vi "Create User UI.vi"() -> ()   [LabVIEW 2016, in "LV-Data.PGSQL.lvclass"]
uses:
  LV-Data.PGSQL.lvclass
  LV-Data/Typedefs/Operation--enum.ctl
  <userlib>/_OpenG.lib/numeric/numeric.llb/Random Number Within Range - DBL__ogtk.vi
  <vilib>/ErrorRing/Error Ring.xnode
  LV-Data/LV-Data.lvclass
panel:
  in  "Delete Permission":bool
  out "Selected User (inst)":string
  in  "Permissions":i32(listbox)
  in  "Give data write permission":bool
  in  "Delete user (inst)":bool
  in  "Users":i32(listbox)
  out "new password":string
  out "new user (inst) name":string
  in  "path to object in table":string
  in  "new password":string
  in  "Create user (inst)":bool
  in  "generate random password?":bool
  in  "new user (inst) name":string
  in  "STOP":bool
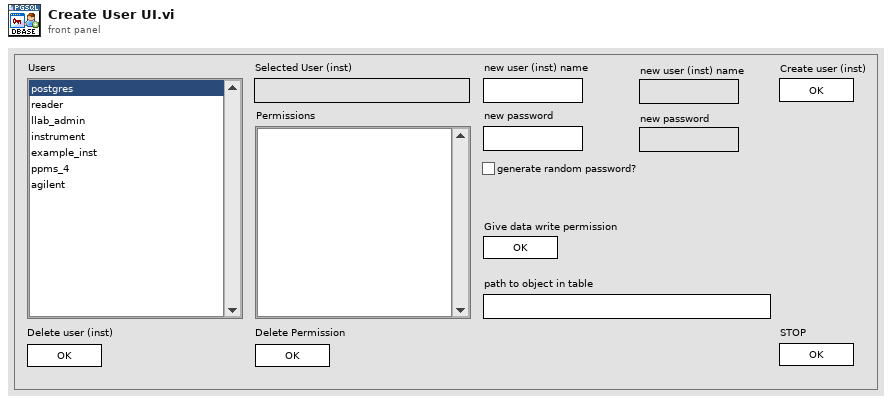
[diagram p1: front panel]
types:
  T1 = enum32{"Invalid", "Standard", "Closed", "Hidden", "Minimized", "Maximized"}
  T2 = enum32{"invalid app kind", "Development System", "Run Time System", "Student Edition", "Embedded LabVIEW", "Evaluation", "Custom"}
  T3 = typedef "LV-Data.lvclass/Operation--enum.ctl" = enum16{"Read", "Write", "Write + Append"}
  T4 = cluster{"Core":cluster{"Current VI Reference":refnum<vi>, "Close Panel on Exit?":bool}, "user":string, "password":string, "path to something in table":string, "new instrument name":string, "names already taken":string[], "Data.PG":refnum<class "LV-Data.PGSQL.lvclass">, "Selected instrument":string, "Selected inst privileges":string[], "Selected inst privileges names":string[], "Selected privilege":string}
  T5 = cluster{"Current VI Reference":refnum<vi>, "Close Panel on Exit?":bool}
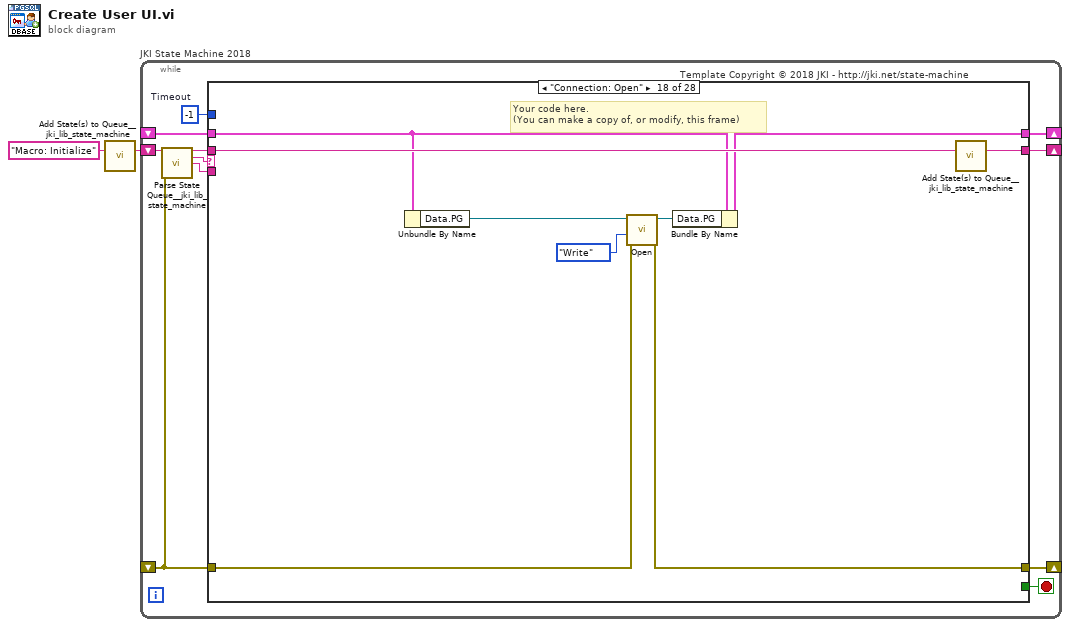
[diagram p0: block diagram]
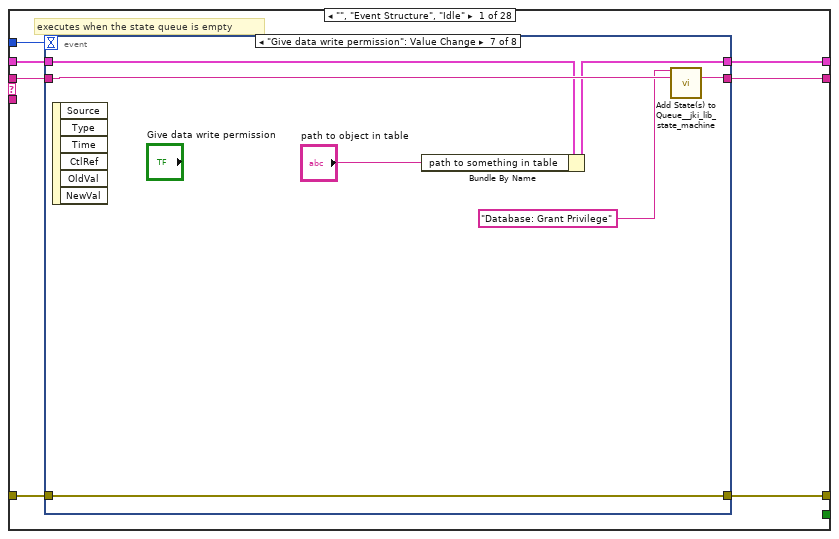
[diagram p2: hidden frame]
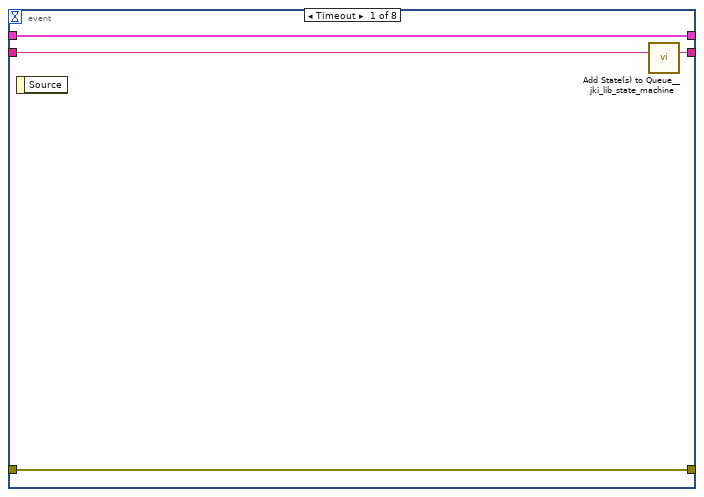
[diagram p3: hidden frame]
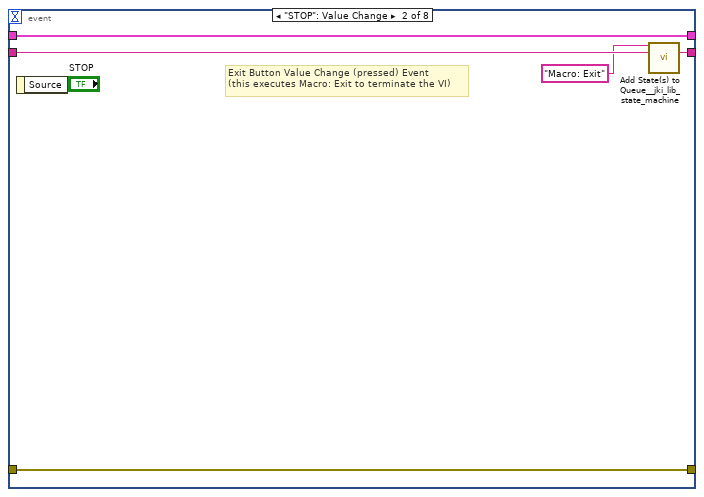
[diagram p4: hidden frame]
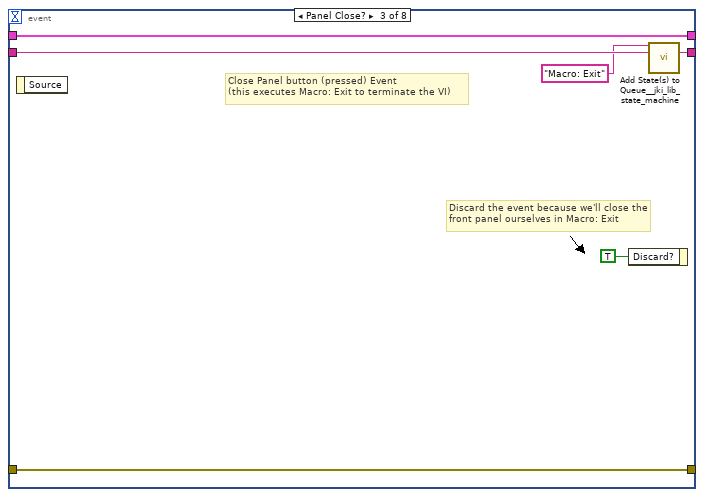
[diagram p5: hidden frame]
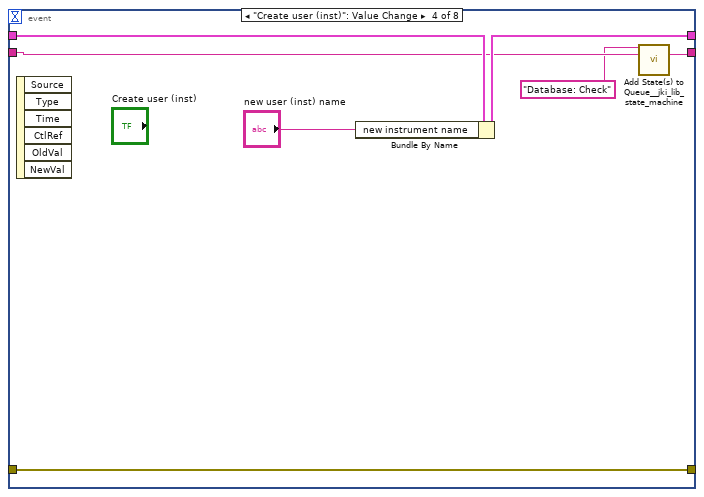
[diagram p6: hidden frame]
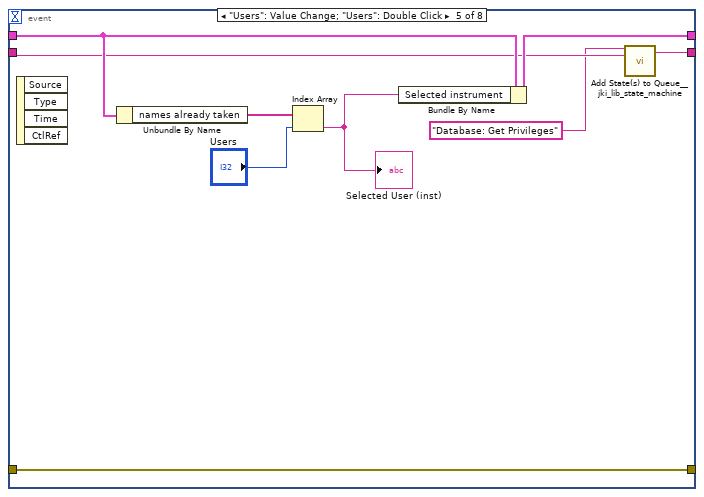
[diagram p7: hidden frame]
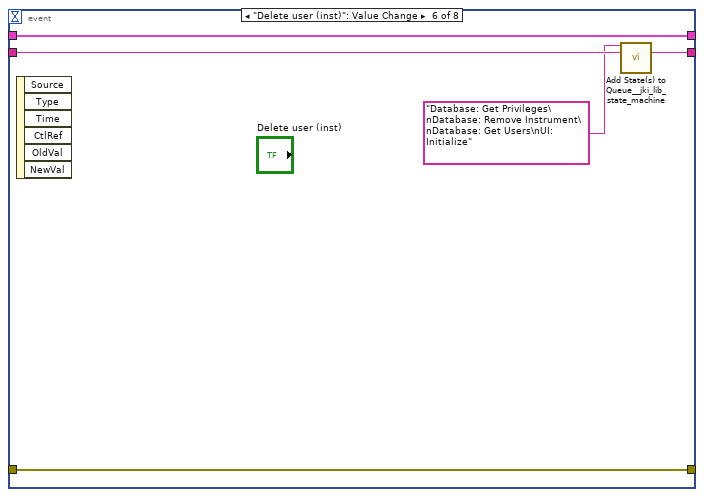
[diagram p8: hidden frame]
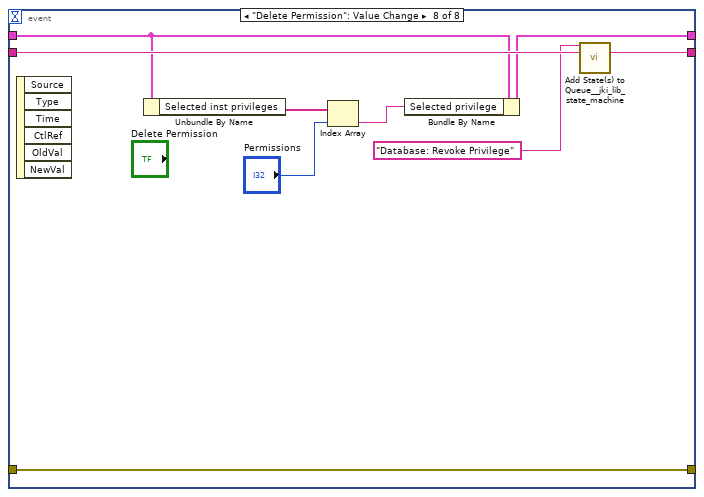
[diagram p9: hidden frame]
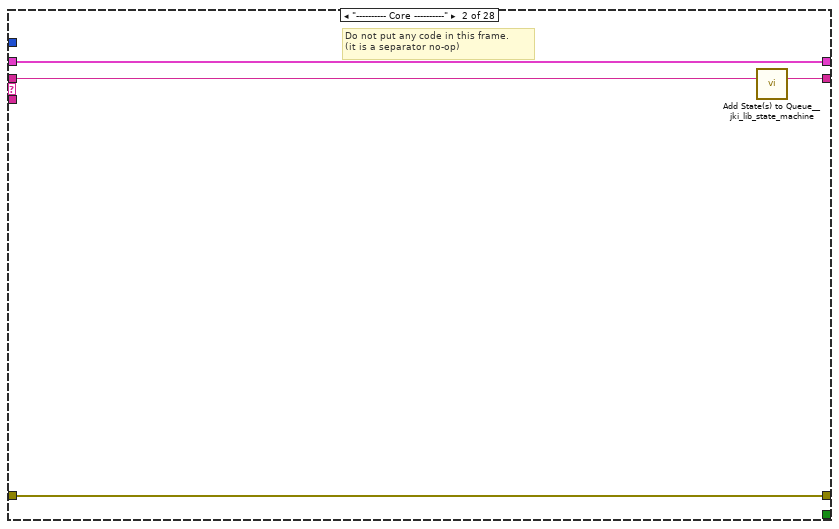
[diagram p10: hidden frame]
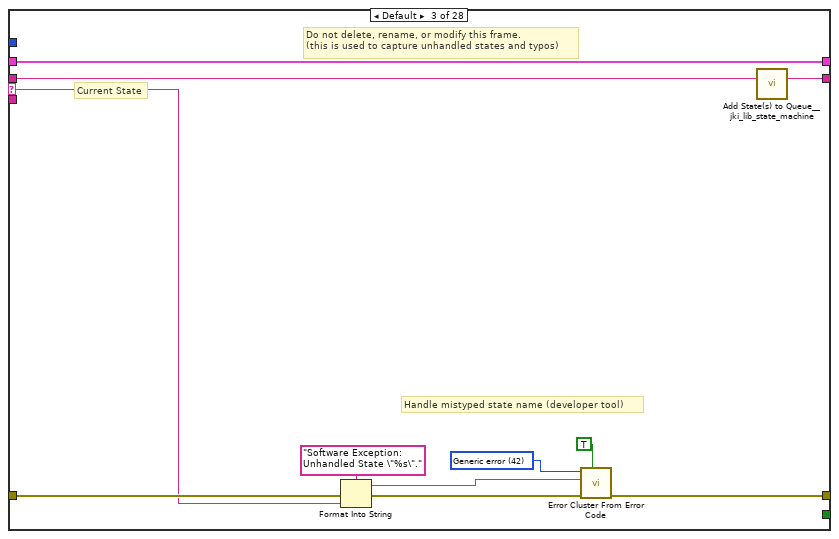
[diagram p11: hidden frame]
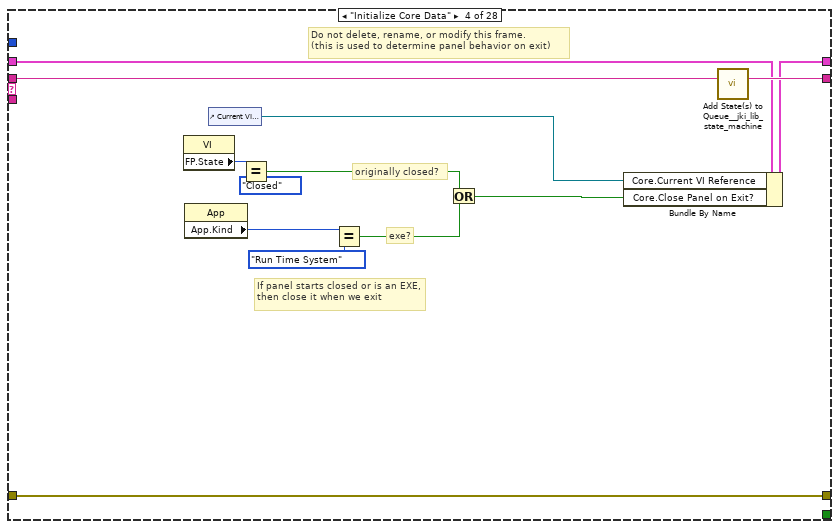
[diagram p12: hidden frame]
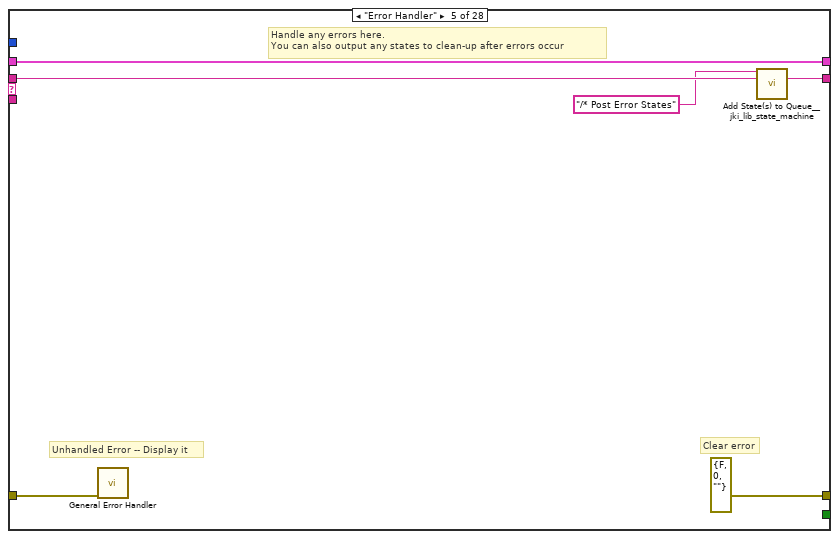
[diagram p13: hidden frame]
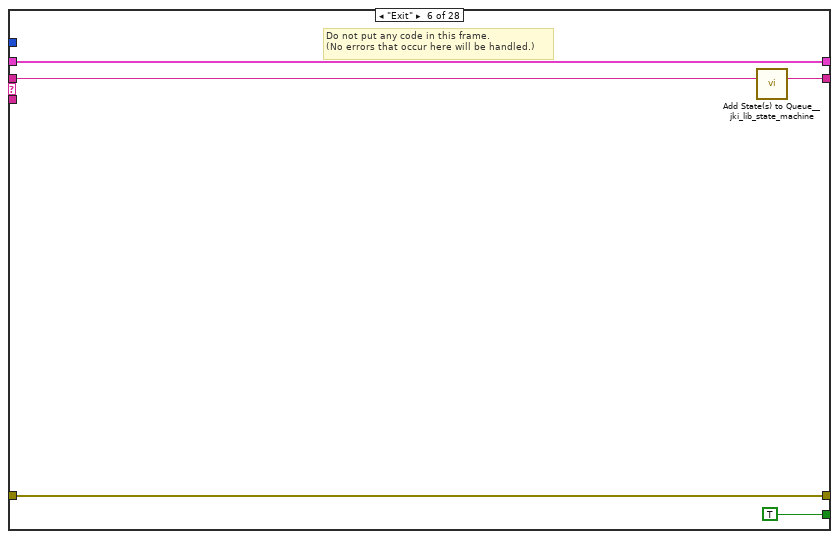
[diagram p14: hidden frame]
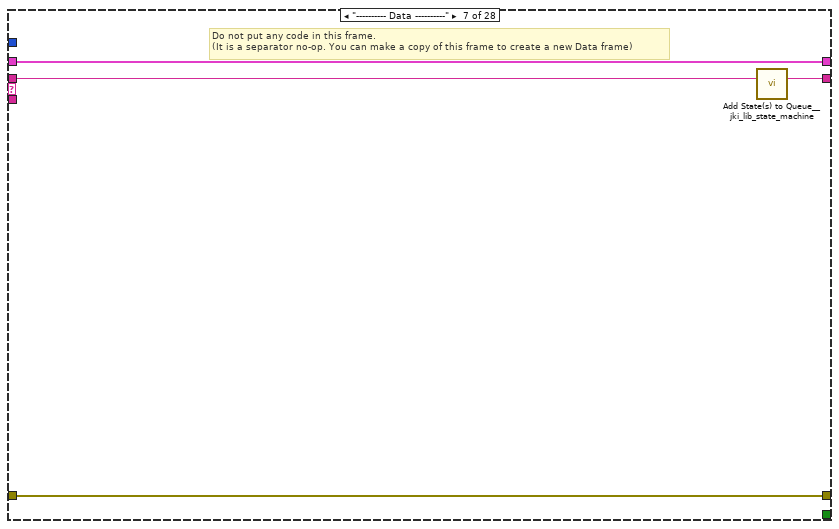
[diagram p15: hidden frame]
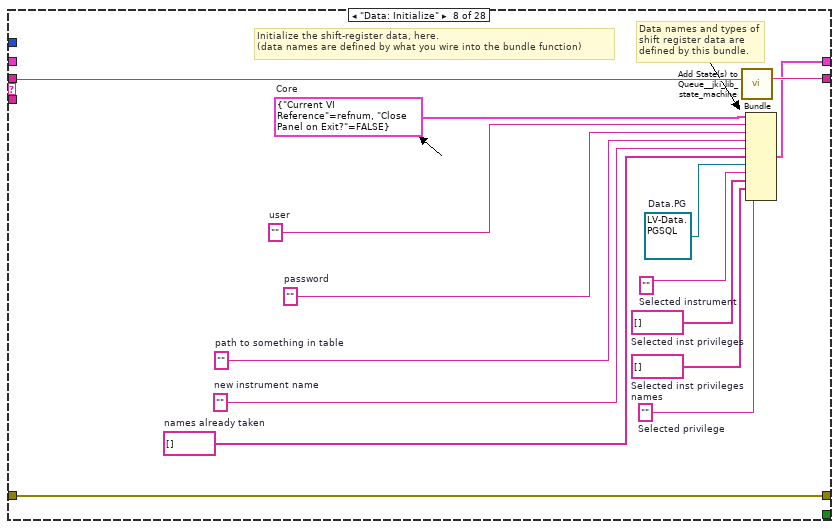
[diagram p16: hidden frame]
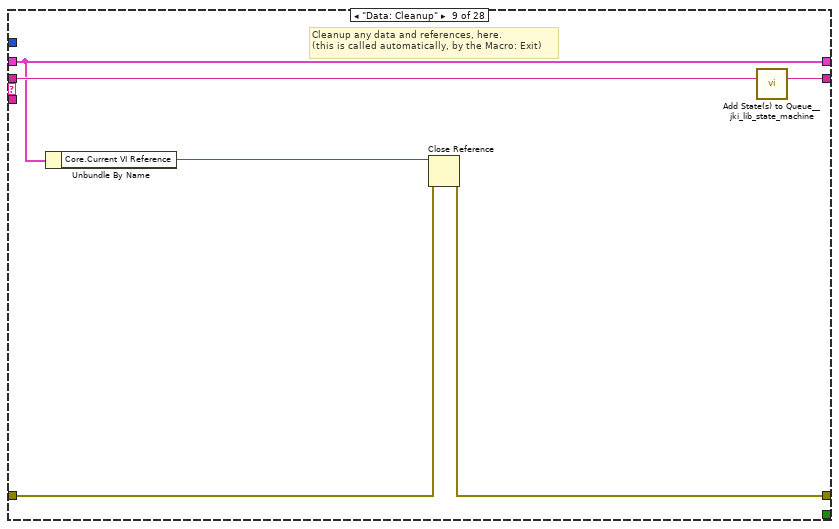
[diagram p17: hidden frame]
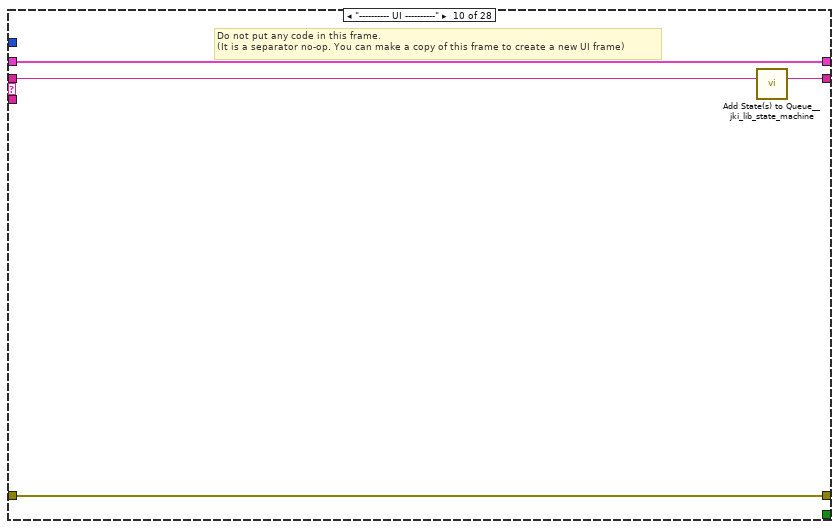
[diagram p18: hidden frame]
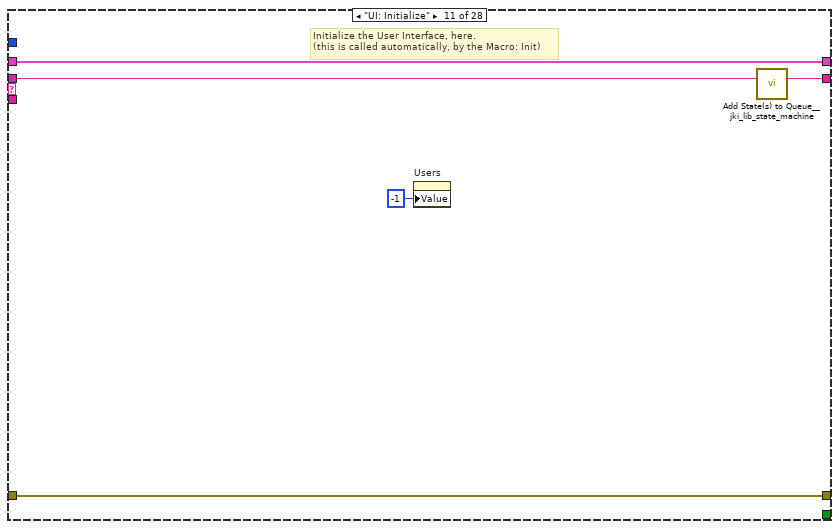
[diagram p19: hidden frame]
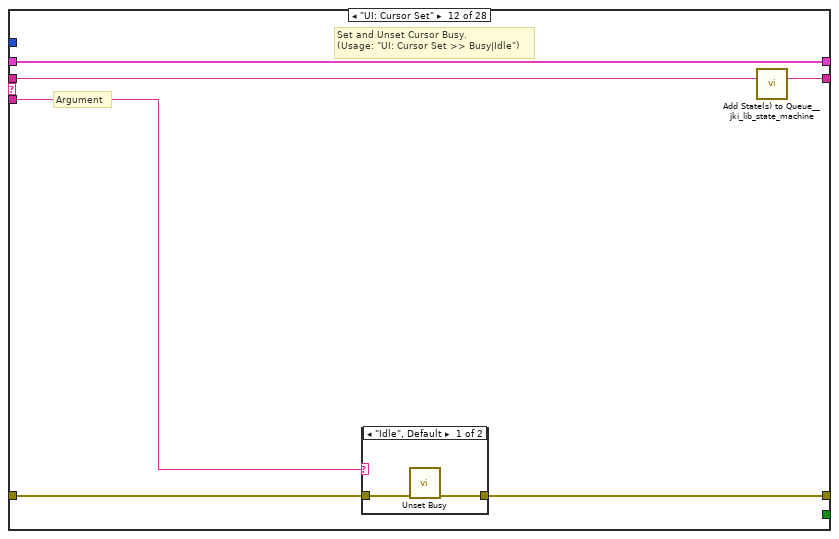
[diagram p20: hidden frame]
diagram:
  n1 = call <vilib>:"Add State(s) to Queue__jki_lib_state_machine.vi"("State(s) in (\"\")"="Macro: Initialize") -> ("States Out"=w2:string)  [unwired: 14 in]
  n2 = while "JKI State Machine 2018" {
    shift-right: [w6] -> _
    shift-left: _ -> [w5]
    shift-right: [w9] -> _
    shift-left: _ -> [w3]
    shift-right: [w8] -> _
    shift-left: w2 -> [w10]
    stop <- w7 stop-if-true
    w4 = -1  # Timeout
    # "Template Copyright © 2018 JKI - http://jki.net/state-machine"
    n3 = call <vilib>:"Parse State Queue__jki_lib_state_machine.vi"("State Queue"=w10, "Error In (no error)"=w3) -> ("Remaining States"=w12:string, "Current State"=w13:string, "Arguments"=w11:string)  [unwired: 11 in]
    n4 = case shown="\"Connection: Open\"" w13 {
      selector: w13 -> [_ _ w77 _ _ _ _ _ _ _ _ _ _ _ _ _ _ _ _ _ _ _ _ _ _ _ _ _]
      tunnel: w12 -> [w20 w76 w81 w100 w106 w111 w115 w130 w136 w140 w145 w151 w162 w231 w236 w247 w251 w260 w266 w270 w279 w291 w326 w340 w353 w368 w378 w408]
      tunnel: w11 -> [_ _ _ _ _ _ _ _ _ _ _ w146 w156 _ _ _ _ _ _ _ _ _ _ _ _ _ _ _]
      tunnel: w5 -> [w18 w73 w79 w93 w103 w109 w112 _ w131 w137 w143 w149 w158 w228 w233 w244 w248 w257 w264 w267 w272 w283 w314 w330 w344 w362 w370 w402]
      tunnel: [w17 w74 w83 w97 errorcluster {"status"=FALSE, "code"=0, "source"=""} ("error out") w108 w113 w128 w132 w138 w142 w147 w159 w229 w234 w245 w249 w253 w261 w268 w274 w281 w322 w337 w345 w354 w372 w399] -> w9
      tunnel: w3 -> [w16 w74 w82 w97 w102 w108 w113 w128 w133 w138 w142 w148 w160 w229 w234 w245 w249 w254 w262 w268 w275 _ w321 w338 w346 w355 w371 w403]
      tunnel: [w19 w75 w80 w99 w105 w110 w114 w129 w135 w139 w144 w150 w161 w230 w235 w246 w250 w259 w265 w269 w278 w290 w325 w339 w352 w367 w377 w407] -> w8
      tunnel: [_ _ _ _ _ TRUE _ _ _ _ _ _ _ _ _ _ _ _ _ _ _ _ _ _ _ _ _ _] -> w7
      tunnel: [w15 w73 w79 w98 w103 w109 w112 w123 w131 w137 w143 w149 w158 w228 w233 w244 w248 w258 w264 w267 w276 w283 w313 w329 w343 w361 w369 w401] -> w6
      tunnel: w4 -> [w14 _ _ _ _ _ _ _ _ _ _ _ _ _ _ _ _ _ _ _ _ _ _ _ _ _ _ _]
      frame "", "Event Structure", "Idle" {
        # "executes when the state queue is empty"
        n5 = event shown="[6] \"Give data write permission\": Value Change" {
          selector: _ -> [_ _ _ _ _ _ _ _]
          dyn-events: _ -> [_ _ _ _ _ _ _ _]
          timeout: w14 -> [_ _ _ _ _ _ _ _]
          tunnel: w20 -> [w24 w29 w35 w38 w44 w53 w62 w71]
          tunnel: [w23 w28 w34 w39 w45 w54 w63 w70] -> w19
          tunnel: w18 -> [w21 w26 w32 w42 w48 w55 w57 w65]
          tunnel: [w22 w27 w33 w37 w51 w56 w61 w72] -> w17
          tunnel: w16 -> [w22 w27 w33 w37 w51 w56 w61 w72]
          tunnel: [w21 w26 w32 w41 w47 w55 w59 w68] -> w15
          event Timeout {
            n6 = event-data() -> ()  [unwired: 1 in, 1 out]
            n7 = call <vilib>:"Add State(s) to Queue__jki_lib_state_machine.vi"("State(s) in (\"\")"=w24) -> ("States Out"=w23:string)  [unwired: 14 in]
          }
          event "STOP": Value Change {
            # "Exit Button Value Change (pressed) Event\n(this executes Macro: Exit to terminate the VI)"
            n8 = event-data() -> ()  [unwired: 1 in, 1 out]
            n9 = call <vilib>:"Add State(s) to Queue__jki_lib_state_machine.vi"("State(s) in Front (\"\")"="Macro: Exit", "State(s) in (\"\")"=w29) -> ("States Out"=w28:string)  [unwired: 13 in]
          }
          event Panel Close? {
            # "Discard the event because we'll close the front panel ourselves in Macro: Exit"
            # "Close Panel button (pressed) Event\n(this executes Macro: Exit to terminate the VI)"
            n10 = event-data() -> ()  [unwired: 1 in, 1 out]
            n11 = event-data("Discard?"=TRUE) -> ()  [unwired: 1 in, 1 out]
            n12 = call <vilib>:"Add State(s) to Queue__jki_lib_state_machine.vi"("State(s) in Front (\"\")"="Macro: Exit", "State(s) in (\"\")"=w35) -> ("States Out"=w34:string)  [unwired: 13 in]
          }
          event "Create user (inst)": Value Change {
            n13 = event-data() -> ()  [unwired: 1 in, 6 out]
            n14 = Bundle By Name(cluster=w42, "new instrument name"="new user (inst) name") -> (w41:T4)
            n15 = call <vilib>:"Add State(s) to Queue__jki_lib_state_machine.vi"("State(s) in Front (\"\")"="Database: Check" ("State(s) in Front (\"\")"), "State(s) in (\"\")"=w38) -> ("States Out"=w39:string)  [unwired: 13 in]
          }
          event "Users": Value Change; "Users": Double Click {
            n16 = event-data() -> ()  [unwired: 1 in, 4 out]
            n17 = Unbundle By Name(w48) -> ("names already taken"=w50:string[])
            n18 = Index Array(array=w50, index="Users") -> (element=w46:string)
            "Selected User (inst)" <- w46
            n19 = Bundle By Name(cluster=w48, "Selected instrument"=w46) -> (w47:T4)
            n20 = call <vilib>:"Add State(s) to Queue__jki_lib_state_machine.vi"("State(s) in Front (\"\")"="Database: Get Privileges" ("State(s) in Front (\"\")"), "State(s) in (\"\")"=w44) -> ("States Out"=w45:string)  [unwired: 13 in]
          }
          event "Delete user (inst)": Value Change {
            n21 = event-data() -> ()  [unwired: 1 in, 6 out]
            n22 = call <vilib>:"Add State(s) to Queue__jki_lib_state_machine.vi"("State(s) in Front (\"\")"="Database: Get Privileges\nDatabase: Remove Instrument\nDatabase: Get Users\nUI: Initialize" ("State(s) in Front (\"\")"), "State(s) in (\"\")"=w53) -> ("States Out"=w54:string)  [unwired: 13 in]
          }
          event "Give data write permission": Value Change {
            n23 = event-data() -> ()  [unwired: 1 in, 6 out]
            n24 = Bundle By Name(cluster=w57, "path to something in table"="path to object in table") -> (w59:T4)
            n25 = call <vilib>:"Add State(s) to Queue__jki_lib_state_machine.vi"("State(s) in Front (\"\")"="Database: Grant Privilege" ("State(s) in Front (\"\")"), "State(s) in (\"\")"=w62) -> ("States Out"=w63:string)  [unwired: 13 in]
          }
          event "Delete Permission": Value Change {
            n26 = event-data() -> ()  [unwired: 1 in, 6 out]
            n27 = Unbundle By Name(w65) -> ("Selected inst privileges"=w64:string[])
            n28 = Index Array(array=w64, index="Permissions") -> (element=w67:string)
            n29 = Bundle By Name(cluster=w65, "Selected privilege"=w67) -> (w68:T4)
            n30 = call <vilib>:"Add State(s) to Queue__jki_lib_state_machine.vi"("State(s) in Front (\"\")"="Database: Revoke Privilege" ("State(s) in Front (\"\")"), "State(s) in (\"\")"=w71) -> ("States Out"=w70:string)  [unwired: 13 in]
          }
        }
      }
      frame "---------- Core ----------" {
        # "Do not put any code in this frame.\n(it is a separator no-op)"
        n31 = call <vilib>:"Add State(s) to Queue__jki_lib_state_machine.vi"("State(s) in (\"\")"=w76) -> ("States Out"=w75:string)  [unwired: 14 in]
      }
      frame Default {
        w86 = 42 items=["No error", "Argument error", "Memory is full", "Out of zone", "End of file", "File already open", "Generic file I/O error", "File not found", "File permission error", "Disk is full", "Duplicate path", "Too many files open", "System feature not enabled", "Resource file not found", "Cannot add resource", "Resource not found", "Image not found", "Image memory error", "Pen does not exist", "Config type invalid", "Config token not found", "Config parse error", "Config memory error", "Bad external code format", "Bad external code offset", "External code not present", "Null window", "Destroy window error", "Null menu", "Print aborted", "Bad print record", "Print driver error", "Windows error during printing", "Memory error during printing", "Print dialog error", "Generic print error", "Invalid device refnum", "Device not found", "Device parameter error", "Device unit error", "Cannot open device", "Device call aborted", "Generic error", "Cancelled by user", "Object ID too low", "Object ID too high", "Object not in heap", "Unknown heap", "Unknown object (invalid DefProc)", "Unknown object (DefProc not in table)", "Message out of range", "Invalid (null) method", "Unknown message", "Manager call not supported", "Bad address", "Network operation in progress", "Network operation timed out", "Connection is busy", "Network attribute not supported", "Network error", "Address in use", "System out of memory", "Connection aborted", "Connection refused", "Not connected", "Already connected", "Connection closed", "Initialization error (interapplication manager)", "Bad occurrence", "Wait on unbound occurrence handler", "Occurrence queue overflow", "Datalog type conflict", "Unused", "Unrecognized type (interapplication manager)", "Memory corrupt", "Failed to make temporary DLL", "Old CIN version", "Drag socket not found", "Failed to load drop-object", "Failed to register OLE object", "Failed to release OLE object", "Format specifier type mismatch", "Unknown format specifier", "Too few format specifiers", "Too many format specifiers", "Scan failed", "Newer CIN version", "Error converting to variant", "Runtime menu error", "Password tampered", "Variant attribute not found", "Incompatible variant data type", "Event data is not available", "Event Store is not present", "Occurrence is not found", "Event Queue is not created", "Event info is not available", "Refnum passed is NULL", "Error retrieving Class GUID", "Error retrieving CoClass GUID", "Error retrieving TypeLib GUID.", "Bad built application magic bytes.", "Specific driver is different from the specific driver associated with the Logical Name.", "There is no session opened to the class driver.", "Max Error", "MAX - Error with config objects", "MAX - Error loading configuration", "MAX - Group not supported"]
        # "Current State"
        # "Do not delete, rename, or modify this frame.\n(this is used to capture unhandled states and typos)"
        # "Handle mistyped state name (developer tool)"
        n32 = Format Into String(format string="Software Exception: Unhandled State \"%s\"." ("message"), error in=w82, w77) -> (resulting string=w85:string, error out=w84:errorcluster)  [unwired: 1 in]
        n33 = call <vilib>:"Error Cluster From Error Code.vi"("show call chain? (False)"=TRUE, "error in (no error)"=w84, "error message (\"\")"=w85, "error code (0)"=w86) -> ("error out"=w83:errorcluster)  [unwired: 5 in]
        n34 = call <vilib>:"Add State(s) to Queue__jki_lib_state_machine.vi"("State(s) in (\"\")"=w81) -> ("States Out"=w80:string)  [unwired: 14 in]
      }
      frame "Initialize Core Data" {
        # "Do not delete, rename, or modify this frame.\n(this is used to determine panel behavior on exit)"
        # "originally closed?"
        # "exe?"
        # "If panel starts closed or is an EXE, then close it when we exit"
        n35 = property class="VI"() -> ("FP.State"=w90:T1)  [unwired: 2 in, 2 out]
        n36 = property class="App"() -> ("App.Kind"=w96:T2)  [unwired: 2 in, 2 out]
        n37 = control-ref of="Current VI Reference"() -> (w91:refnum<vi>)
        n38 = Equal?(x=w90, y=T1."Closed" ("Front Panel Window:State")) -> (x = y?=w88:bool)
        n39 = Equal?(x=w96, y=T2."Run Time System" ("Application:Kind")) -> (x = y?=w94:bool)
        n40 = Or(x=w88, y=w94) -> (x .or. y?=w92:bool)
        n41 = Bundle By Name(cluster=w93, "Core.Current VI Reference"=w91, "Core.Close Panel on Exit?"=w92) -> (w98:T4)
        n42 = call <vilib>:"Add State(s) to Queue__jki_lib_state_machine.vi"("State(s) in (\"\")"=w100) -> ("States Out"=w99:string)  [unwired: 14 in]
      }
      frame "Error Handler" {
        # "Unhandled Error -- Display it"
        # "Handle any errors here.\nYou can also output any states to clean-up after errors occur"
        # "Clear error"
        n43 = call <vilib>:"General Error Handler.vi"("error in (no error)"=w102) -> ()  [unwired: 10 in, 5 out]
        n44 = call <vilib>:"Add State(s) to Queue__jki_lib_state_machine.vi"("State(s) in Front (\"\")"="/* Post Error States", "State(s) in (\"\")"=w106) -> ("States Out"=w105:string)  [unwired: 13 in]
      }
      frame "Exit" {
        # "Do not put any code in this frame.\n(No errors that occur here will be handled.)"
        n45 = call <vilib>:"Add State(s) to Queue__jki_lib_state_machine.vi"("State(s) in (\"\")"=w111) -> ("States Out"=w110:string)  [unwired: 14 in]
      }
      frame "---------- Data ----------" {
        # "Do not put any code in this frame.\n(It is a separator no-op. You can make a copy of this frame to create a new Data frame)"
        n46 = call <vilib>:"Add State(s) to Queue__jki_lib_state_machine.vi"("State(s) in (\"\")"=w115) -> ("States Out"=w114:string)  [unwired: 14 in]
      }
      frame "Data: Initialize" {
        w116 = ""  # password
        w117 = ""  # Selected privilege
        w118 = string[] []  # Selected inst privileges names
        w119 = ""  # user
        w120 = string[] []  # Selected inst privileges
        w121 = ""  # Selected instrument
        w122 = refnum<class "LV-Data.PGSQL.lvclass"> refnum  # Data.PG
        w125 = string[] []  # names already taken
        w126 = ""  # new instrument name
        w127 = ""  # path to something in table
        w124 = T5 {"Current VI Reference"=refnum, "Close Panel on Exit?"=FALSE}  # Core
        # "Data names and types of shift register data are defined by this bundle."
        # "Initialize the shift-register data, here.\n(data names are defined by what you wire into the bundle function)"
        n47 = call <vilib>:"Add State(s) to Queue__jki_lib_state_machine.vi"("State(s) in (\"\")"=w130) -> ("States Out"=w129:string)  [unwired: 14 in]
        n48 = Bundle("Core"=w124, "user"=w119, "password"=w116, "path to something in table"=w127, "new instrument name"=w126, "names already taken"=w125, "Data.PG"=w122, "Selected instrument"=w121, "Selected inst privileges"=w120, "Selected inst privileges names"=w118, "Selected privilege"=w117) -> (w123:T4)  [unwired: 1 in]
      }
      frame "Data: Cleanup" {
        # "Cleanup any data and references, here.\n(this is called automatically, by the Macro: Exit)"
        n49 = Unbundle By Name(w131) -> ("Core.Current VI Reference"=w134:refnum<vi>)
        n50 = Close Reference(reference=w134, error in (no error)=w133) -> (error out=w132:errorcluster)
        n51 = call <vilib>:"Add State(s) to Queue__jki_lib_state_machine.vi"("State(s) in (\"\")"=w136) -> ("States Out"=w135:string)  [unwired: 14 in]
      }
      frame "---------- UI ----------" {
        # "Do not put any code in this frame.\n(It is a separator no-op. You can make a copy of this frame to create a new UI frame)"
        n52 = call <vilib>:"Add State(s) to Queue__jki_lib_state_machine.vi"("State(s) in (\"\")"=w140) -> ("States Out"=w139:string)  [unwired: 14 in]
      }
      frame "UI: Initialize" {
        # "Initialize the User Interface, here.\n(this is called automatically, by the Macro: Init)"
        n53 = property on="Users" class="LstBox (strict)"("Value"=-1 ("Users")) -> ()  [unwired: 2 in, 2 out]
        n54 = call <vilib>:"Add State(s) to Queue__jki_lib_state_machine.vi"("State(s) in (\"\")"=w145) -> ("States Out"=w144:string)  [unwired: 14 in]
      }
      frame "UI: Cursor Set" {
        # "Argument"
        # "Set and Unset Cursor Busy.\n(Usage: \"UI: Cursor Set >> Busy|Idle\")"
        n55 = case shown="\"Idle\", Default" w146 {
          tunnel: w148 -> [w153 w155]
          tunnel: [w152 w154] -> w147
          frame "Idle", Default {
            n56 = call <vilib>:"Unset Busy.vi"("error in (no error)"=w153) -> ("error out"=w152:errorcluster)  [unwired: 10 in]
          }
          frame "Busy" {
            n57 = call <vilib>:"Set Busy.vi"("error in (no error)"=w155) -> ("error out"=w154:errorcluster)  [unwired: 9 in, 1 out]
          }
        }
        n58 = call <vilib>:"Add State(s) to Queue__jki_lib_state_machine.vi"("State(s) in (\"\")"=w151) -> ("States Out"=w150:string)  [unwired: 14 in]
      }
      frame "UI: Front Panel State" {
        # "Argument"
        # "Set Front Panel Open or Closed\n(Usage: \"UI: Front Panel State >> Open|Close\")"
        n59 = Unbundle By Name(w158) -> ("Core.Current VI Reference"=w157:refnum<vi>)
        n60 = case shown="\"Minimize\", \"Minimized\"" w156 {
          tunnel: w160 -> [w168 w183 w194 w207 w220]
          tunnel: [w170 w184 w196 w209 w222] -> w159
          tunnel: w157 -> [w169 w181 w195 w208 w221]
          frame "Open", "Standard", Default {
            w163 = T1."Standard" ("State")
            n61 = property class="VI"(reference=w169, error in=w168) -> (reference out=w166:refnum<vi>, error out=w167:errorcluster, "FP.State"=w165:T1)
            n62 = Not Equal?(x=w165, y=w163) -> (x != y?=w164:bool)
            n63 = case shown="True" w164 {
              tunnel: [w174 w176] -> w170
              tunnel: w167 -> [w173 w176]
              tunnel: w166 -> [w172 _]
              tunnel: w163 -> [w171 _]
              frame True {
                n64 = invoke class="VI" method="FP.Open"(reference=w172, error in=w173, "Activate"=TRUE, "State"=w171) -> (error out=w174:errorcluster)  [unwired: 1 in, 4 out]
              }
              frame False {
              }
            }
          }
          frame "Close", "Closed" {
            n65 = property class="VI"(reference=w181, error in=w183) -> (reference out=w180:refnum<vi>, error out=w182:errorcluster, "FP.State"=w178:T1)
            n66 = Not Equal?(x=w178, y=T1."Closed" ("Front Panel Window:State")) -> (x != y?=w177:bool)
            n67 = case shown="True" w177 {
              tunnel: [w185 w188] -> w184
              tunnel: w182 -> [w185 w187]
              tunnel: w180 -> [_ w186]
              frame False {
              }
              frame True {
                n68 = invoke class="VI" method="FP.Close"(reference=w186, error in=w187) -> (error out=w188:errorcluster)  [unwired: 1 in, 2 out]
              }
            }
          }
          frame "Hidden", "Hide" {
            w189 = T1."Hidden" ("State")
            n69 = property class="VI"(reference=w195, error in=w194) -> (reference out=w192:refnum<vi>, error out=w193:errorcluster, "FP.State"=w191:T1)
            n70 = Not Equal?(x=w191, y=w189) -> (x != y?=w190:bool)
            n71 = case shown="True" w190 {
              tunnel: [w200 w201] -> w196
              tunnel: w193 -> [w199 w201]
              tunnel: w192 -> [w198 _]
              tunnel: w189 -> [w197 _]
              frame True {
                n72 = invoke class="VI" method="FP.Open"(reference=w198, error in=w199, "State"=w197) -> (error out=w200:errorcluster)  [unwired: 2 in, 4 out]
              }
              frame False {
              }
            }
          }
          frame "Minimize", "Minimized" {
            w202 = T1."Minimized" ("State")
            n73 = property class="VI"(reference=w208, error in=w207) -> (reference out=w205:refnum<vi>, error out=w206:errorcluster, "FP.State"=w204:T1)
            n74 = Not Equal?(x=w204, y=w202) -> (x != y?=w203:bool)
            n75 = case shown="True" w203 {
              tunnel: [w213 w214] -> w209
              tunnel: w206 -> [w212 w214]
              tunnel: w205 -> [w211 _]
              tunnel: w202 -> [w210 _]
              frame True {
                n76 = invoke class="VI" method="FP.Open"(reference=w211, error in=w212, "State"=w210) -> (error out=w213:errorcluster)  [unwired: 2 in, 4 out]
              }
              frame False {
              }
            }
          }
          frame "Maximize", "Maximized" {
            w215 = T1."Maximized" ("State")
            n77 = property class="VI"(reference=w221, error in=w220) -> (reference out=w218:refnum<vi>, error out=w219:errorcluster, "FP.State"=w217:T1)
            n78 = Not Equal?(x=w217, y=w215) -> (x != y?=w216:bool)
            n79 = case shown="True" w216 {
              tunnel: [w226 w227] -> w222
              tunnel: w219 -> [w225 w227]
              tunnel: w218 -> [w224 _]
              tunnel: w215 -> [w223 _]
              frame True {
                n80 = invoke class="VI" method="FP.Open"(reference=w224, error in=w225, "State"=w223) -> (error out=w226:errorcluster)  [unwired: 2 in, 4 out]
              }
              frame False {
              }
            }
          }
        }
        n81 = call <vilib>:"Add State(s) to Queue__jki_lib_state_machine.vi"("State(s) in (\"\")"=w162) -> ("States Out"=w161:string)  [unwired: 14 in]
      }
      frame "---------- Macro ----------" {
        # "Do not put any code in this frame.\n(It is a separator no-op. You can make a copy of this frame to create a new Macro frame)"
        n82 = call <vilib>:"Add State(s) to Queue__jki_lib_state_machine.vi"("State(s) in (\"\")"=w231) -> ("States Out"=w230:string)  [unwired: 14 in]
      }
      frame "Macro: Initialize" {
        w232 = "Data: Initialize\nInitialize Core Data\nUI: Initialize\nUI: Front Panel State >> Open\nConnection: Open\nDatabase: Get Users"  # Data: Initialize Initialize Core Data UI: Initialize UI: Front Panel State >> Open Connection: Open Database: Get Users
        # "Initialization Macro\n(This is called once, when the VI starts)"
        n83 = call <vilib>:"Add State(s) to Queue__jki_lib_state_machine.vi"("State(s) in Front (\"\")"=w232, "State(s) in (\"\")"=w236) -> ("States Out"=w235:string)  [unwired: 13 in]
      }
      frame "Macro: Exit" {
        # "Exit Macro\n(This is called once, when the VI exits)"
        n84 = Unbundle By Name(w244) -> ("Core.Close Panel on Exit?"=w243:bool)
        n85 = Select(t="UI: Front Panel State >> Close", s=w243, f="") -> (s? t:f=w240:string)
        n86 = property on="new password" class="Str"("Text.Text"="") -> ()  [unwired: 2 in, 2 out]
        n87 = call <vilib>:"Add State(s) to Queue__jki_lib_state_machine.vi"("State(s) in (\"\")"=w240, "State(s) at Back (\"\")"="Connection: Close\nData: Cleanup\nExit") -> ("States Out"=w238:string)  [unwired: 13 in]
        n88 = call <vilib>:"Add State(s) to Queue__jki_lib_state_machine.vi"("State(s) in Front (\"\")"=w238, "State(s) in (\"\")"=w247) -> ("States Out"=w246:string)  [unwired: 13 in]
      }
      frame "---------- Connection ----------" {
        # "Template Separator\n(You can make a copy of, or modify, this frame)"
        n89 = call <vilib>:"Add State(s) to Queue__jki_lib_state_machine.vi"("State(s) in (\"\")"=w251) -> ("States Out"=w250:string)  [unwired: 14 in]
      }
      frame "Connection: Open" {
        # "Your code here.\n(You can make a copy of, or modify, this frame)"
        n90 = Unbundle By Name(w257) -> ("Data.PG"=w255:refnum<class "LV-Data.PGSQL.lvclass">)
        n91 = call-dynamic "Open.vi"("error in (no error)"=w254, "Operation"=Operation--enum."Write", "Data.PG in"=w255) -> ("error out"=w253:errorcluster, "Data.PG out"=w256:refnum<class "LV-Data.PGSQL.lvclass">)  [unwired: 7 in]
        n92 = Bundle By Name(cluster=w257, "Data.PG"=w256) -> (w258:T4)
        n93 = call <vilib>:"Add State(s) to Queue__jki_lib_state_machine.vi"("State(s) in (\"\")"=w260) -> ("States Out"=w259:string)  [unwired: 14 in]
      }
      frame "Connection: Close" {
        # "Your code here.\n(You can make a copy of, or modify, this frame)"
        n94 = Unbundle By Name(w264) -> ("Data.PG"=w263:refnum<class "LV-Data.PGSQL.lvclass">)
        n95 = call-dynamic "Close.vi"("error in (no error)"=w262, "Data.PG in"=w263) -> ("error out"=w261:errorcluster)  [unwired: 8 in, 1 out]
        n96 = call <vilib>:"Add State(s) to Queue__jki_lib_state_machine.vi"("State(s) in (\"\")"=w266) -> ("States Out"=w265:string)  [unwired: 14 in]
      }
      frame "---------- Database ----------" {
        # "Template Separator\n(You can make a copy of, or modify, this frame)"
        n97 = call <vilib>:"Add State(s) to Queue__jki_lib_state_machine.vi"("State(s) in (\"\")"=w270) -> ("States Out"=w269:string)  [unwired: 14 in]
      }
      frame "Database: Get Users" {
        # "Template Separator\n(You can make a copy of, or modify, this frame)"
        n98 = Unbundle By Name(w272) -> ("Data.PG"=w277:refnum<class "LV-Data.PGSQL.lvclass">)
        n99 = call "Get Users.vi"("error in (no error)"=w275, "Data.PG"=w277) -> ("error out"=w274:errorcluster, "Users"=w273:string[], "Data.PG out"=w271:refnum<class "LV-Data.PGSQL.lvclass">)  [unwired: 7 in]
        n100 = property on="Users" class="LstBox (strict)"("Item Names"=w273) -> ()  [unwired: 2 in, 2 out]
        n101 = Bundle By Name(cluster=w272, "Data.PG"=w271, "names already taken"=w273) -> (w276:T4)
        n102 = call <vilib>:"Add State(s) to Queue__jki_lib_state_machine.vi"("State(s) in (\"\")"=w279) -> ("States Out"=w278:string)  [unwired: 14 in]
      }
      frame "Database: Check" {
        # "Template Separator\n(You can make a copy of, or modify, this frame)"
        n103 = Unbundle By Name(w283) -> ("names already taken"=w289:string[], "new instrument name"=w282:string)
        n104 = call <userlib>:"Search or Split String__ogtk.vi"("search string/char (-)"=" ", "string"=w282) -> ("offset after match"=w285:i32)  [unwired: 1 in, 2 out]
        n105 = Increment(x=w285) -> (x+1=w284:i32)
        n106 = for {
          tunnel: w289 -> [w309] mode=indexing
          tunnel: w282 -> [w308]
          shift-right: [w307] -> w288
          shift-left: w284 -> [w306]
          n107 = Equal?(x=w309, y=w308) -> (x = y?=w303:bool)
          n108 = Select(t=1, s=w303, f=0) -> (s? t:f=w302:i32)
          n109 = Add(x=w302, y=w306) -> (x+y=w307:i32)
        }
        n110 = Equal To 0?(x=w288) -> (x = 0?=w287:bool)
        n111 = case shown="False" w287 {
          tunnel: ["" "Database: Create User"] -> w280
          tunnel: [w292 w299] -> w281
          frame False {
            n112 = xnode "Error Ring"() -> ("error out"=w292:errorcluster)
          }
          frame True {
            n113 = xnode "Error Ring"() -> ("error out"=w299:errorcluster)
          }
        }
        n114 = call <vilib>:"Add State(s) to Queue__jki_lib_state_machine.vi"("State(s) in Front (\"\")"=w280, "State(s) in (\"\")"=w291) -> ("States Out"=w290:string)  [unwired: 13 in]
      }
      frame "Database: Create User" {
        # "Template Separator\n(You can make a copy of, or modify, this frame)"
        n115 = Unbundle By Name(w314) -> ("Data.PG"=w324:refnum<class "LV-Data.PGSQL.lvclass">, "new instrument name"=w310:string)
        "new user (inst) name" <- w310
        n116 = call-poly <userlib>:"Random Number Within Range__ogtk.vi"("High"=i64 9223372036854775807 ("upper bound (100)"), "Low"=0) -> ("Random Number"=w317:dbl)  [unwired: 3 in]
        n117 = Number To Hexadecimal String(2:w317) -> (0:w315:string)  [unwired: 1 in]
        n118 = Select(t=w315, s="generate random password?", f="new password") -> (s? t:f=w311:string)
        "new password" <- w311
        n119 = call "Create User.vi"("error in (no error)"=w321, "new user password"=w311, "new user name"=w310, "Data.PGSQL in"=w324) -> ("error out"=w322:errorcluster, "Data.PGSQL out"=w312:refnum<class "LV-Data.PGSQL.lvclass">)  [unwired: 6 in]
        n120 = Bundle By Name(cluster=w314, "Data.PG"=w312) -> (w313:T4)
        n121 = call <vilib>:"Add State(s) to Queue__jki_lib_state_machine.vi"("State(s) in Front (\"\")"="Database: Get Users" ("State(s) in Front (\"\")"), "State(s) in (\"\")"=w326) -> ("States Out"=w325:string)  [unwired: 13 in]
      }
      frame "Database: Grant Privilege" {
        # "Template Separator\n(You can make a copy of, or modify, this frame)"
        n122 = Unbundle By Name(w330) -> ("Data.PG"=w333:refnum<class "LV-Data.PGSQL.lvclass">, "path to something in table"=w332:string, "Selected instrument"=w334:string)
        n123 = call "Parse Path Name.vi"("PG Path"=w332) -> ("Table path"=w331:string)  [unwired: 10 in, 4 out]
        n124 = Format Into String(format string="GRANT INSERT ON %s TO %s", w331, w334) -> (resulting string=w336:string)  [unwired: 2 in, 1 out]
        n125 = call "Execute SQL.vi"("error in"=w338, "SQL"=w336, "Data.PG"=w333) -> ("error out"=w337:errorcluster, "Data.PG out"=w328:refnum<class "LV-Data.PGSQL.lvclass">)  [unwired: 6 in, 1 out]
        n126 = Bundle By Name(cluster=w330, "Data.PG"=w328) -> (w329:T4)
        n127 = call <vilib>:"Add State(s) to Queue__jki_lib_state_machine.vi"("State(s) in Front (\"\")"="Database: Get Privileges" ("State(s) in Front (\"\")"), "State(s) in (\"\")"=w340) -> ("States Out"=w339:string)  [unwired: 13 in]
      }
      frame "Database: Revoke Privilege" {
        # "Template Separator\n(You can make a copy of, or modify, this frame)"
        n128 = Unbundle By Name(w344) -> ("Data.PG"=w348:refnum<class "LV-Data.PGSQL.lvclass">, "Selected privilege"=w350:string, "Selected instrument"=w349:string)
        n129 = Format Into String(format string="REVOKE INSERT ON %s FROM %s;", w350, w349) -> (resulting string=w347:string)  [unwired: 2 in, 1 out]
        n130 = call "Execute SQL.vi"("error in"=w346, "SQL"=w347, "Data.PG"=w348) -> ("error out"=w345:errorcluster, "Data.PG out"=w342:refnum<class "LV-Data.PGSQL.lvclass">)  [unwired: 6 in, 1 out]
        n131 = Bundle By Name(cluster=w344, "Data.PG"=w342) -> (w343:T4)
        n132 = call <vilib>:"Add State(s) to Queue__jki_lib_state_machine.vi"("State(s) in Front (\"\")"="Database: Get Privileges" ("State(s) in Front (\"\")"), "State(s) in (\"\")"=w353) -> ("States Out"=w352:string)  [unwired: 13 in]
      }
      frame "Database: Get Privileges" {
        # "Template Separator\n(You can make a copy of, or modify, this frame)"
        n133 = Unbundle By Name(w362) -> ("Data.PG"=w366:refnum<class "LV-Data.PGSQL.lvclass">, "Selected instrument"=w359:string)
        n134 = Format Into String(format string="SELECT table_name FROM information_schema.role_table_grants WHERE (grantee = '%s' and privilege_type ='INSERT');", w359) -> (resulting string=w360:string)  [unwired: 2 in, 1 out]
        n135 = call "Execute SQL.vi"("error in"=w355, "SQL"=w360, "Data.PG"=w366) -> ("error out"=w354:errorcluster, "Result"=w364:string[][], "Data.PG out"=w356:refnum<class "LV-Data.PGSQL.lvclass">)  [unwired: 6 in]
        n136 = Transpose 2D Array(2D array=w364) -> (transposed array=w363:string[][])
        n137 = Index Array(array=w363) -> (element=w358:string[])  [unwired: 2 in]
        n138 = Bundle By Name(cluster=w362, "Data.PG"=w356, "Selected inst privileges"=w358) -> (w361:T4)
        n139 = call <vilib>:"Add State(s) to Queue__jki_lib_state_machine.vi"("State(s) in Front (\"\")"="Database: Privileges Paths to Names" ("State(s) in Front (\"\")"), "State(s) in (\"\")"=w368) -> ("States Out"=w367:string)  [unwired: 13 in]
      }
      frame "Database: Privileges Paths to Names" {
        # "Template Separator\n(You can make a copy of, or modify, this frame)"
        n140 = Unbundle By Name(w370) -> ("Data.PG"=w374:refnum<class "LV-Data.PGSQL.lvclass">, "Selected inst privileges"=w375:string[])
        n141 = for {
          tunnel: w375 -> [w383] mode=indexing
          tunnel: [w385] -> w373 mode=concatenating
          tunnel: w374 -> [w384]
          shift-right: [w379] -> w372
          shift-left: w371 -> [w380]
          n142 = Search/Split String(string=w383, search string/char (-)="index" ("true string")) -> (offset of match=w381:i32)  [unwired: 1 in, 2 out]
          n143 = case shown="-1" w381 {
            tunnel: w383 -> [w388 w395]
            tunnel: [w387 w392] -> w385
            tunnel: w384 -> [_ w397]
            tunnel: w380 -> [w386 w391]
            tunnel: [w386 w390] -> w379
            frame 0, Default {
              n144 = Build Array(w388) -> (w387:string[])
            }
            frame -1 {
              n145 = Format Into String(format string="SELECT name FROM table_index WHERE path='%s';", w395) -> (resulting string=w396:string)  [unwired: 2 in, 1 out]
              n146 = call "Execute SQL.vi"("error in"=w391, "SQL"=w396, "Data.PG"=w397) -> ("error out"=w390:errorcluster, "Result"=w389:string[][])  [unwired: 6 in, 1 out]
              n147 = Transpose 2D Array(2D array=w389) -> (transposed array=w394:string[][])
              n148 = Index Array(array=w394, index (row)=0) -> (element=w392:string[])  [unwired: 1 in]
            }
          }
        }
        n149 = Bundle By Name(cluster=w370, "Selected inst privileges names"=w373) -> (w369:T4)
        n150 = property on="Permissions" class="LstBox (strict)"("Item Names"=w373, "Value"=-1 ("Permissions")) -> ()  [unwired: 2 in, 2 out]
        n151 = call <vilib>:"Add State(s) to Queue__jki_lib_state_machine.vi"("State(s) in (\"\")"=w378) -> ("States Out"=w377:string)  [unwired: 14 in]
      }
      frame "Database: Remove Instrument" {
        # "Template Separator\n(You can make a copy of, or modify, this frame)"
        n152 = Unbundle By Name(w402) -> ("Data.PG"=w406:refnum<class "LV-Data.PGSQL.lvclass">, "Selected inst privileges"=w405:string[], "Selected instrument"=w404:string)
        n153 = case shown="Default" w404 {
          selector: w404 -> [w410 _]
          tunnel: [w415 w428] -> w399
          tunnel: w406 -> [w414 w427]
          tunnel: w405 -> [w418 _]
          tunnel: w403 -> [w411 _]
          tunnel: [w409 w427] -> w400
          frame Default {
            n154 = for {
              tunnel: w418 -> [w424] mode=indexing
              tunnel: w410 -> [w423]
              tunnel: w411 -> [w419]
              tunnel: [w420] -> w412
              shift-right: [w421] -> w413
              shift-left: w414 -> [w422]
              n155 = Format Into String(format string="REVOKE INSERT ON %s FROM %s;", w424, w423) -> (resulting string=w426:string)  [unwired: 2 in, 1 out]
              n156 = call "Execute SQL.vi"("error in"=w419, "SQL"=w426, "Data.PG"=w422) -> ("error out"=w420:errorcluster, "Data.PG out"=w421:refnum<class "LV-Data.PGSQL.lvclass">)  [unwired: 6 in, 1 out]
            }
            n157 = Format Into String(format string="REVOKE instrument FROM %s;\nDROP ROLE %s;", w410, w410) -> (resulting string=w417:string)  [unwired: 2 in, 1 out]
            n158 = call "Execute SQL.vi"("error in"=w412, "SQL"=w417, "Data.PG"=w413) -> ("error out"=w415:errorcluster, "Data.PG out"=w409:refnum<class "LV-Data.PGSQL.lvclass">)  [unwired: 6 in, 1 out]
          }
          frame "instrument", "llab_admin", "postgres", "reader" {
            n159 = xnode "Error Ring"() -> ("error out"=w428:errorcluster)
          }
        }
        n160 = Bundle By Name(cluster=w402, "Data.PG"=w400) -> (w401:T4)
        n161 = call <vilib>:"Add State(s) to Queue__jki_lib_state_machine.vi"("State(s) in (\"\")"=w408) -> ("States Out"=w407:string)  [unwired: 14 in]
      }
    }
  }
